vi "Parse Port (Tx-UDP-CommPort).vi"(8 "error in":errorcluster, 11 "node in":refnum<k20>) -> (0 "error out":errorcluster, 3 "tx udp comm port out":T1 {"Parameters"."Parameter"."encoding" items=["BNR", "BCD", "Discrete"]})   [LabVIEW 2020, in "AIM ARINC 664 Import.lvlib"]
uses:
  AIM ARINC 664 Import.lvlib
  _typedefs/port_tx_udp_comm.ctl
  _typedefs/frame_parameter.ctl
  _typedefs/frame_parameter_definition.ctl
  Shared/Encoding (Arinc664).ctl
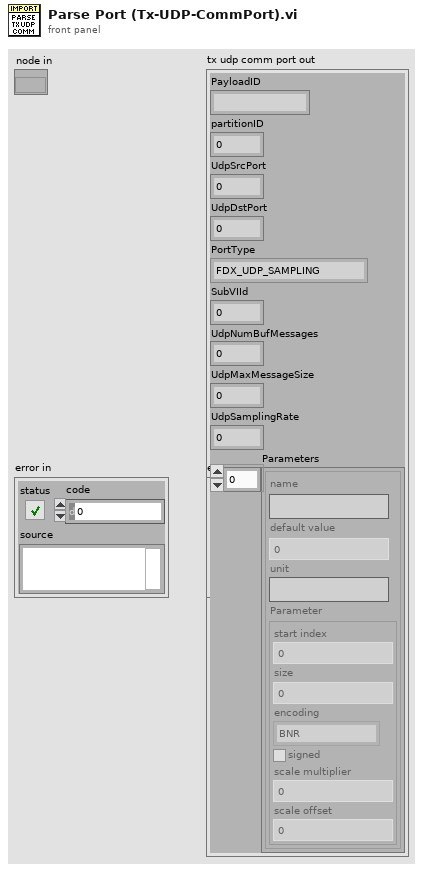
[diagram p1: front panel]
types:
  T1 = typedef "AIM ARINC 664 Import.lvlib/port_tx_udp_comm.ctl" = cluster{"PayloadID":string, "partitionID":u8, "UdpSrcPort":u16, "UdpDstPort":u16, "PortType":enum16{"FDX_UDP_SAMPLING", "FDX_UDP_QUEUING"}, "SubVIId":u32, "UdpNumBufMessages":u32, "UdpMaxMessageSize":u32, "UdpSamplingRate":u32, "Parameters":T2[]}
  T2 = typedef "AIM ARINC 664 Import.lvlib/frame_parameter.ctl" = cluster{"name":string, "default value":dbl, "unit":string, "Parameter":T3}
  T3 = typedef "AIM ARINC 664 Import.lvlib/frame_parameter_definition.ctl" = cluster{"start index":i32, "size":i32, "encoding":T4, "signed":bool, "scale multiplier":dbl, "scale offset":dbl}
  T4 = typedef "Encoding (Arinc664).ctl" = u16
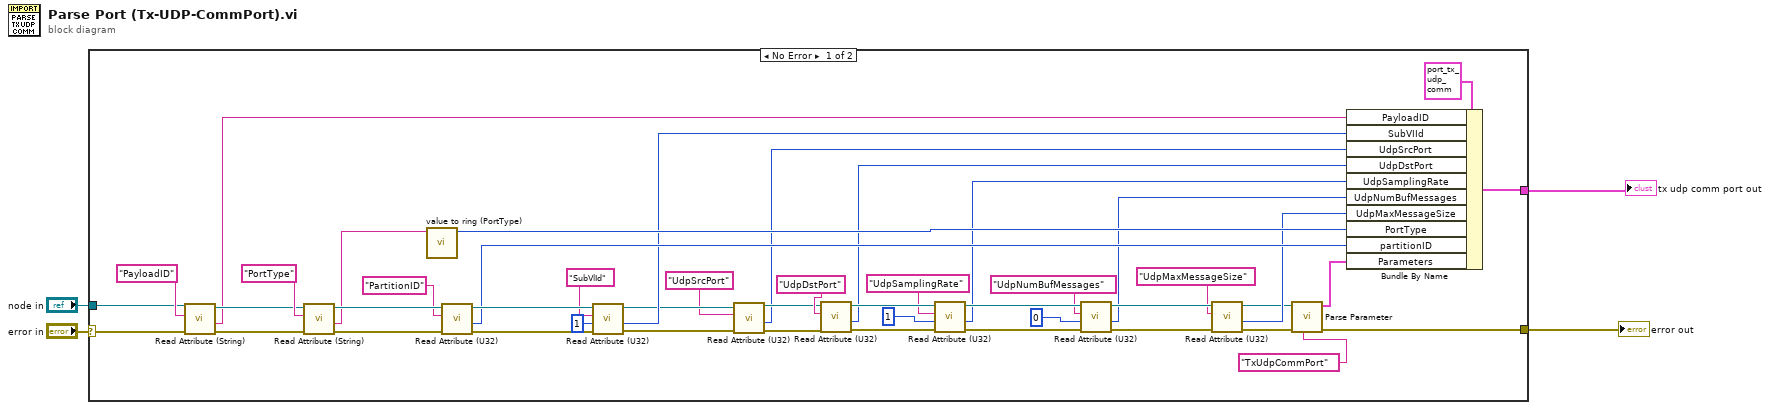
[diagram p0: block diagram]
diagram:
  n1 = case shown="No Error" "error in" {
    selector: "error in" -> [w7 w52]
    tunnel: "node in" -> [w9 _]
    tunnel: [w13 w52] -> w3
    tunnel: [w51 _] -> w1
    frame No Error {
      n2 = call "Read Attribute (String).vi"("error in"=w7, "Attribute Name"="PayloadID" ("Name"), "node in"=w9) -> ("error out"=w6:errorcluster, "value"=w5:string, "node out"=w8:refnum<k20>)  [unwired: 6 in]
      n3 = call "Read Attribute (String).vi"("error in"=w6, "Attribute Name"="PortType" ("Name"), "node in"=w8) -> ("error out"=w48:errorcluster, "value"=w42:string, "node out"=w50:refnum<k20>)  [unwired: 6 in]
      n4 = call "value to ring (PortType).vi"("value"=w42) -> ("PortType"=w41:enum16{"FDX_UDP_SAMPLING", "FDX_UDP_QUEUING"})  [unwired: 10 in]
      n5 = call "Read Attribute (U32).vi"("error in"=w48, "Attribute Name"="PartitionID" ("Tag Name"), "node in"=w50) -> ("error out"=w47:errorcluster, "value"=w40:u32, "node out"=w49:refnum<k20>)  [unwired: 6 in]
      n6 = call "Read Attribute (U32).vi"("error in"=w47, "default"=u32 1, "Attribute Name"="SubVlId" ("Tag Name"), "node in"=w49) -> ("error out"=w23:errorcluster, "value"=w39:u32, "node out"=w24:refnum<k20>)  [unwired: 5 in]
      n7 = call "Read Attribute (U32).vi"("error in"=w23, "Attribute Name"="UdpSrcPort" ("Tag Name"), "node in"=w24) -> ("error out"=w22:errorcluster, "value"=w19:u32, "node out"=w21:refnum<k20>)  [unwired: 6 in]
      n8 = call "Read Attribute (U32).vi"("error in"=w22, "Attribute Name"="UdpDstPort" ("Tag Name"), "node in"=w21) -> ("error out"=w37:errorcluster, "value"=w25:u32, "node out"=w38:refnum<k20>)  [unwired: 6 in]
      n9 = call "Read Attribute (U32).vi"("error in"=w37, "default"=u32 1, "Attribute Name"="UdpSamplingRate" ("Tag Name"), "node in"=w38) -> ("error out"=w34:errorcluster, "value"=w27:u32, "node out"=w33:refnum<k20>)  [unwired: 5 in]
      n10 = call "Read Attribute (U32).vi"("error in"=w34, "default"=u32 0, "Attribute Name"="UdpNumBufMessages" ("Tag Name"), "node in"=w33) -> ("error out"=w36:errorcluster, "value"=w30:u32, "node out"=w35:refnum<k20>)  [unwired: 5 in]
      n11 = call "Read Attribute (U32).vi"("error in"=w36, "Attribute Name"="UdpMaxMessageSize" ("Tag Name"), "node in"=w35) -> ("error out"=w14:errorcluster, "value"=w31:u32, "node out"=w15:refnum<k20>)  [unwired: 6 in]
      n12 = call "Parse Parameter.vi"("error text in"="TxUdpCommPort", "error in"=w14, "node in"=w15) -> ("error out"=w13:errorcluster, "parametesrs"=w12:T2[])  [unwired: 7 in]
      n13 = Bundle By Name(cluster=T1 {"PayloadID"="", "partitionID"=0, "UdpSrcPort"=0, "UdpDstPort"=0, "PortType"=enum."FDX_UDP_SAMPLING", "SubVIId"=0, "UdpNumBufMessages"=0, "UdpMaxMessageSize"=0, "UdpSamplingRate"=0, "Parameters"=[]} ("session_tx_generic"), "PayloadID"=w5, "SubVIId"=w39, "UdpSrcPort"=w19, "UdpDstPort"=w25, "UdpSamplingRate"=w27, "UdpNumBufMessages"=w30, "UdpMaxMessageSize"=w31, "PortType"=w41, "partitionID"=w40, "Parameters"=w12) -> (w51:T1)
    }
    frame Error {
    }
  }
  "error out" <- w3
  "tx udp comm port out" <- w1
